vi "3. vision影像選顏色範圍.vi"() -> ()   [LabVIEW 2014]
uses:
  <vilib>/vision/driver/NI_Vision_Acquisition_Software.lvlib
  <vilib>/vision/NI_Vision_Development_Module.lvlib
panel:
  out "選擇範圍":T1(plugin-control)
  in  "亮度":cluster{"Min":i32, "Max":i32}(slide)={"Min"=60, "Max"=157} scale=0.0..255.0
  in  "飽和度":cluster{"Min":i32, "Max":i32}(slide)={"Min"=0, "Max"=42} scale=0.0..255.0
  in  "色相":cluster{"Min":i32, "Max":i32}(slide)={"Min"=67, "Max"=120} scale=0.0..255.0
  out "顯示錯誤":errorcluster
  out "影像":T1(plugin-control)
  in  "stop":bool
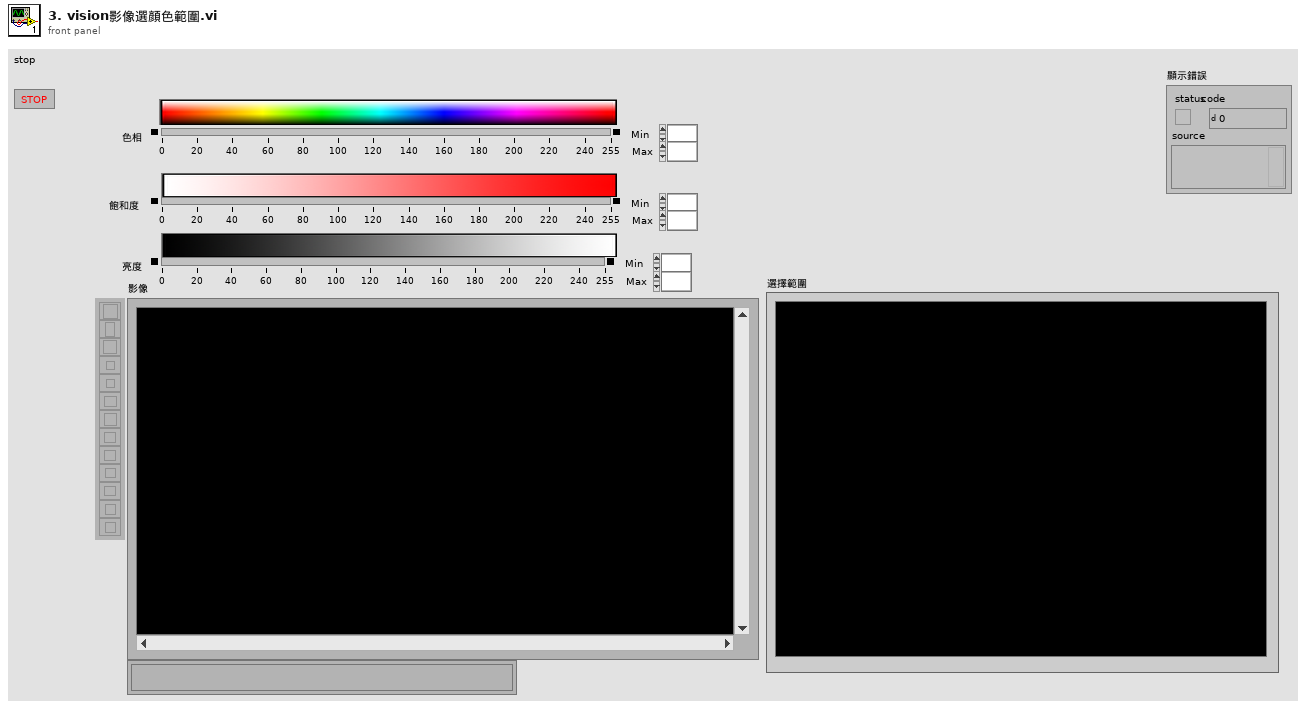
[diagram p1: front panel]
types:
  T1 = typedef "IMAQ Image.ctl" = refnum<image>
  T2 = typedef "Image Type" = u32
  T3 = cluster{"Type":u32, "Version":u32, "Flags":u32, "SerialNumberHigh":u32, "SerialNumberLow":u32, "BusType":u32, "InterfaceName":string, "VendorName":string, "ModelName":string, "CameraFileName":string, "CameraAttributeURL":string}[]
  T4 = cluster{"Type":u32, "Version":u32, "Flags":u32, "SerialNumberHigh":u32, "SerialNumberLow":u32, "BusType":u32, "InterfaceName":string, "VendorName":string, "ModelName":string, "CameraFileName":string, "CameraAttributeURL":string}
  T5 = typedef "IMAQdx.ctl" = refnum<k21>
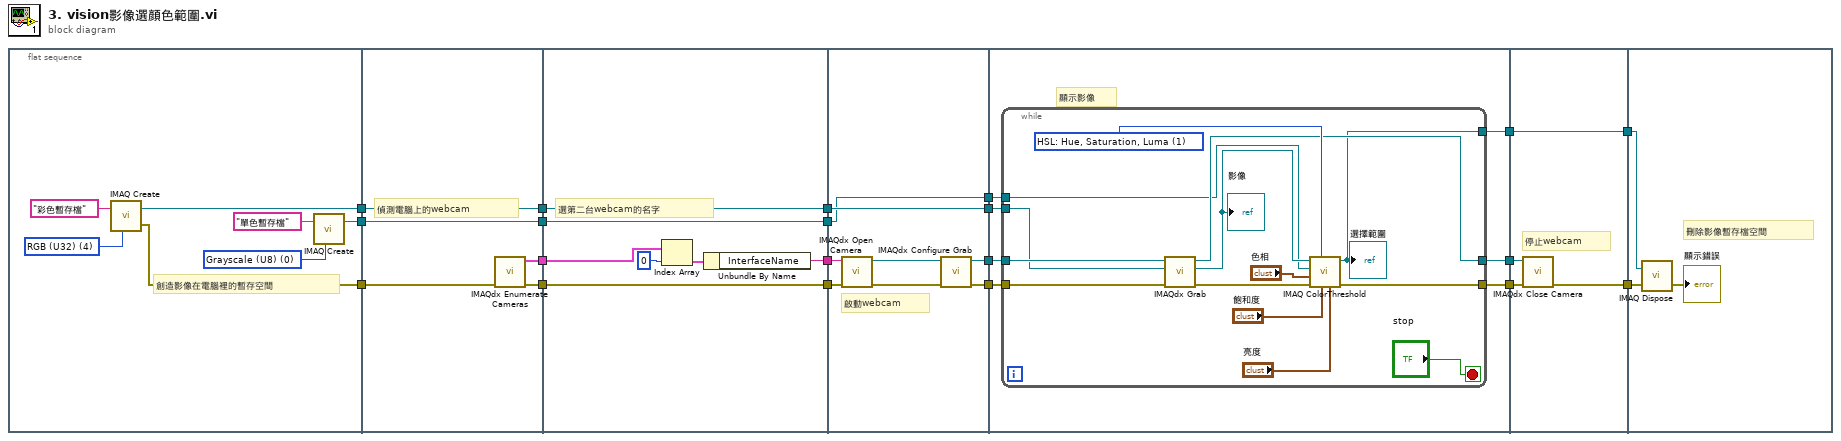
[diagram p0: block diagram]
diagram:
  n1 = flat-sequence {
    tunnel: [w25] -> w14
    tunnel: [w24] -> w13
    tunnel: [w21] -> w4
    tunnel: [w32] -> w20
    tunnel: [w31] -> w15
    tunnel: w14 -> [w31]
    tunnel: w13 -> [w30]
    tunnel: [w29] -> w11
    tunnel: [w28] -> w5
    tunnel: w4 -> [w28]
    tunnel: w20 -> [w37]
    tunnel: [w36] -> w19
    tunnel: [w35] -> w16
    tunnel: w15 -> [w35]
    tunnel: [w34] -> w12
    tunnel: w11 -> [w34]
    tunnel: [w33] -> w6
    tunnel: w5 -> [w33]
    tunnel: w19 -> [w46]
    tunnel: [w45] -> w18
    tunnel: [w44] -> w17
    tunnel: w16 -> [w44]
    tunnel: w12 -> [w43]
    tunnel: [w41] -> w10
    tunnel: [w40] -> w7
    tunnel: w6 -> [w40]
    tunnel: w18 -> [w54]
    tunnel: w17 -> [w53]
    tunnel: w10 -> [w52]
    tunnel: [w51] -> w8
    tunnel: w7 -> [w50]
    tunnel: [w49] -> w3
    tunnel: [w48] -> w2
    tunnel: [w72] -> w9
    tunnel: w8 -> [w71]
    tunnel: w3 -> [w70]
    tunnel: w2 -> [w69]
    tunnel: [w69] -> w1
    tunnel: w9 -> [w75]
    tunnel: w1 -> [w73]
    frame #0 {
      w22 = T2 0 items=["Grayscale (U8)", "Grayscale (I16)", "Grayscale (SGL)", "Complex (CSG)", "RGB (U32)", "HSL (U32)", "RGB (U64)", "Grayscale (U16)"] ("Image Type")
      w27 = T2 4 items=["Grayscale (U8)", "Grayscale (I16)", "Grayscale (SGL)", "Complex (CSG)", "RGB (U32)", "HSL (U32)", "RGB (U64)", "Grayscale (U16)"] ("Image Type")
      # "創造影像在電腦裡的暫存空間"
      n2 = call "IMAQ Create"("Image Name"="彩色暫存檔", "Image Type"=w27) -> ("New Image"=w25:T1, "error out"=w24:errorcluster)  [unwired: 3 in]
      n3 = call "IMAQ Create"("Image Name"="單色暫存檔", "Image Type"=w22) -> ("New Image"=w21:T1)  [unwired: 3 in, 1 out]
    }
    frame #1 {
      # "偵測電腦上的webcam"
      n4 = call <vilib>:"IMAQdx Enumerate Cameras.vi"("error in"=w30) -> ("error out"=w29:errorcluster, "Camera Information Array"=w32:T3)  [unwired: 9 in]
    }
    frame #2 {
      # "選第二台webcam的名字"
      n5 = Index Array(array=w37, index=0) -> (element=w38:T4)
      n6 = Unbundle By Name(w38) -> ("InterfaceName"=w36:string)
    }
    frame #3 {
      # "啟動webcam"
      n7 = call <vilib>:"IMAQdx Open Camera.vi"("error in"=w43, "Session In"=w46) -> ("error out"=w42:errorcluster, "Session Out"=w47:T5)  [unwired: 8 in]
      n8 = call <vilib>:"IMAQdx Configure Grab.vi"("error in"=w42, "Session In"=w47) -> ("error out"=w41:errorcluster, "Session Out"=w45:T5)  [unwired: 8 in]
    }
    frame #4 {
      # "顯示影像"
      n9 = while {
        tunnel: w54 -> [w67]
        tunnel: w53 -> [w66]
        tunnel: w52 -> [w65]
        tunnel: [w59] -> w51
        tunnel: w50 -> [w57]
        tunnel: [w56] -> w49
        tunnel: [w55] -> w48
        stop <- "stop" stop-if-true
        w64 = 1 items=["RGB (Red, Green, Blue)", "HSL: Hue, Saturation, Luma"] ("Threshold Color Mode")
        n10 = call <vilib>:"IMAQdx Grab.vi"("error in"=w65, "Image In"=w66, "Session In"=w67) -> ("error out"=w60:errorcluster, "Image Out"=w58:T1, "Session Out"=w59:T5)  [unwired: 5 in, 1 out]
        "影像" <- w58
        n11 = call "IMAQ ColorThreshold"("Blue or Luma or Val or Inten Range"="亮度", "Green or Sat Range"="飽和度", "Color Mode"=w64, "error in (no error)"=w60, "Red or Hue Range"="色相", "Image Dst"=w57, "Image Src"=w58) -> ("error out"=w56:errorcluster, "Image Dst Out"=w55:T1)  [unwired: 1 in, 2 out]
        "選擇範圍" <- w55
      }
    }
    frame #5 {
      # "停止webcam"
      n12 = call <vilib>:"IMAQdx Close Camera.vi"("error in"=w70, "Session In"=w71) -> ("error out"=w72:errorcluster)  [unwired: 9 in]
    }
    frame #6 {
      # "刪除影像暫存檔空間"
      n13 = call "IMAQ Dispose"("Image"=w73, "error in (no error)"=w75) -> ("error out"=→"顯示錯誤":errorcluster)  [unwired: 4 in]
    }
  }
